vi "HEWH Extract DBL Data.vi"(7 "Full Data (String)":string[][](array[string]), 8 "error in (no error)":errorcluster, 10 "Full Data DBL In":dbl[][](array[numeric]), 11 "UEF Calculated Values Input in":T1 {"Data Indexes"."15 sec after Draw Index" format="%#.2f"; "Data Indexes"."15 sec after Draw Timestamp" format="%#.2f"; "Data Indexes"."Test Start Timestamp" format="%.2f"; "Data Indexes"."Test End Timestamp" format="%.2f"; "Data Indexes"."T0 Timestamp" format="%.2f"; "Data Indexes"."Tsf Timestamp" format="%.2f"; "Data Indexes"."Tsu0 Timestamp" format="%.2f"; "Data Indexes"."Tmax1 Timestamp" format="%.2f"; "Data Indexes"."Draw Index Timestamp" format="%#.2f"; "Data Indexes"."Non-Draw Timestamp" format="%#.2f"; "Data Indexes"."Heating Timestamp" format="%#.2f"; "Data Indexes"."Start Energy (BTU-Gas)" format="%.6f"; "Data Indexes"."Start Watt Hours" format="%.6f"; "Static Data"."V - Volume of Wh (True)" format="%.5f"; "Static Data"."T-Ambinet Nominal (°F)" format="%.5f"; "Static Data"."T-Inlet Setpoint (°F)" format="%.5f"; "Static Data"."T-Wh Setpoint (°F)" format="%.5f"; "Sampled Data"."Qe (Wh)" format="%.5f"; "Sampled Data"."Tau stby2 (hr)" format="%.5f"; "Sampled Data"."Tastby2 (°F)" format="%.5f"; "Sampled Data"."Qf (BTU)" format="%.5f"; "Sampled Data"."Qe (BTU)" format="%.5f"; "Sampled Data"."Tmax1 (°F)" format="%.5f"; "Sampled Data"."T0 (°F)" format="%.5f"; "Sampled Data"."Qr (BTU)" format="%.5f"; "Sampled Data"."T 24(°F)" format="%.5f"; "Sampled Data"."T astby(°F)" format="%.5f"; "Sampled Data"."T tstby(°F)" format="%.5f"; "Sampled Data"."T su0(°F)" format="%.5f"; "Sampled Data"."T suf(°F)" format="%.5f"; "Sampled Data"."Tau stby_1 (hr)" format="%.5f"; "Sampled Data"."Qsuf (BTU)" format="%.5f"; "Sampled Data"."Qsu0 (BTU)" format="%.5f"; "Calculated Values"."Draw Bonus Volume (gal)" format="%.6f"; "Calculated Values"."Adjustment Factor" format="%.6f"; "Calculated Values"."T*avg_del(n-1)" format="%.6f"; "Calculated Values"."T*min(n-1)" format="%.6f"; "Calculated Values"."T*avg_del(n)" format="%.6f"; "Calculated Values"."Vn" format="%.6f"; "Calculated Values"."Qdm (BTU)" format="%.6f"; "Calculated Values"."QHWD (BTU)" format="%.6f"; "Calculated Values"."QHW (BTU)" format="%.6f"; "Calculated Values"."UEF" format="%.6f"; "Calculated Values"."QHW67 (BTU)" format="%.6f"; "Calculated Values"."Qda (BTU)" format="%.6f"; "Calculated Values"."Qd (BTU)" format="%.6f"; "Calculated Values"."Q (BTU)" format="%.6f"; "Calculated Values"."UA (BTU/(hr*F))" format="%.6f"; "Calculated Values"."Qhr (BTU/hr)" format="%.6f"; "Calculated Values"."Qstby (BTU)" format="%.6f"; "Calculated Values"."nu_r" format="%.6f"; "Calculated Values"."CpUEF (BTU/(lb*F))" format="%.6f"; "Calculated Values"."rho_nu (lb/gal)" format="%.6f"; "Calculated Values"."V1- Vol (Gal)" format="%.6f"; "Calculated Values"."M cluster mass removed (lb)" format="%.6f"; "Calculated Values"."Cp theoretical (BTU/(lbm °F))" format="%.6f"; "Calculated Values"."Tin1 - Mean Inlet 1st Cluster (°F)" format="%.6f"; "Calculated Values"."Tdel1-Mean Outlet 1st Cluster(°F)" format="%.6f"; "Calculated Values"."Cp 24 (BTU/(lb*F))" format="%.6f"; "Calculated Values"."Cp standby (BTU/(lb*F))" format="%.6f"; "Calculated Values"."Cp2 (BTU/(lb*F))" format="%.6f"; "Calculated Values"."Cp1 (BTU/(lb*F))" format="%.6f"; "Calculated Values"."rho 24 (lb/gal)" format="%.6f"; "Calculated Values"."rho standby (lb/gal)" format="%.6f"; "Calculated Values"."rho 2 (lb/gal)" format="%.6f"; "Calculated Values"."Density of cold water All (lbm/gal)" format="%#.3g"; "Calculated Values"."CpHW (BTU/(lbm °F))" format="%#.3g"; "Calculated Values"."Density of hot water All (lbm/gal)" format="%#.3g"; "Calculated Values"."Mass of water All (lbm)" format="%#.3f"}) -> (0 "error out":errorcluster, 2 "Full Data DBL Out":dbl[][](array[numeric]), 3 "UEF Calculated Values Input out":T1 {"Data Indexes"."15 sec after Draw Index" format="%#.2f"; "Data Indexes"."15 sec after Draw Timestamp" format="%#.2f"; "Data Indexes"."Test Start Timestamp" format="%.2f"; "Data Indexes"."Test End Timestamp" format="%.2f"; "Data Indexes"."T0 Timestamp" format="%.2f"; "Data Indexes"."Tsf Timestamp" format="%.2f"; "Data Indexes"."Tsu0 Timestamp" format="%.2f"; "Data Indexes"."Tmax1 Timestamp" format="%.2f"; "Data Indexes"."Draw Index Timestamp" format="%#.2f"; "Data Indexes"."Non-Draw Timestamp" format="%#.2f"; "Data Indexes"."Heating Timestamp" format="%#.2f"; "Data Indexes"."Start Energy (BTU-Gas)" format="%.6f"; "Data Indexes"."Start Watt Hours" format="%.6f"; "Static Data"."V - Volume of Wh (True)" format="%.5f"; "Static Data"."T-Ambinet Nominal (°F)" format="%.5f"; "Static Data"."T-Inlet Setpoint (°F)" format="%.5f"; "Static Data"."T-Wh Setpoint (°F)" format="%.5f"; "Sampled Data"."Qe (Wh)" format="%.5f"; "Sampled Data"."Tau stby2 (hr)" format="%.5f"; "Sampled Data"."Tastby2 (°F)" format="%.5f"; "Sampled Data"."Qf (BTU)" format="%.5f"; "Sampled Data"."Qe (BTU)" format="%.5f"; "Sampled Data"."Tmax1 (°F)" format="%.5f"; "Sampled Data"."T0 (°F)" format="%.5f"; "Sampled Data"."Qr (BTU)" format="%.5f"; "Sampled Data"."T 24(°F)" format="%.5f"; "Sampled Data"."T astby(°F)" format="%.5f"; "Sampled Data"."T tstby(°F)" format="%.5f"; "Sampled Data"."T su0(°F)" format="%.5f"; "Sampled Data"."T suf(°F)" format="%.5f"; "Sampled Data"."Tau stby_1 (hr)" format="%.5f"; "Sampled Data"."Qsuf (BTU)" format="%.5f"; "Sampled Data"."Qsu0 (BTU)" format="%.5f"; "Calculated Values"."Draw Bonus Volume (gal)" format="%.6f"; "Calculated Values"."Adjustment Factor" format="%.6f"; "Calculated Values"."T*avg_del(n-1)" format="%.6f"; "Calculated Values"."T*min(n-1)" format="%.6f"; "Calculated Values"."T*avg_del(n)" format="%.6f"; "Calculated Values"."Vn" format="%.6f"; "Calculated Values"."Qdm (BTU)" format="%.6f"; "Calculated Values"."QHWD (BTU)" format="%.6f"; "Calculated Values"."QHW (BTU)" format="%.6f"; "Calculated Values"."UEF" format="%.6f"; "Calculated Values"."QHW67 (BTU)" format="%.6f"; "Calculated Values"."Qda (BTU)" format="%.6f"; "Calculated Values"."Qd (BTU)" format="%.6f"; "Calculated Values"."Q (BTU)" format="%.6f"; "Calculated Values"."UA (BTU/(hr*F))" format="%.6f"; "Calculated Values"."Qhr (BTU/hr)" format="%.6f"; "Calculated Values"."Qstby (BTU)" format="%.6f"; "Calculated Values"."nu_r" format="%.6f"; "Calculated Values"."CpUEF (BTU/(lb*F))" format="%.6f"; "Calculated Values"."rho_nu (lb/gal)" format="%.6f"; "Calculated Values"."V1- Vol (Gal)" format="%.6f"; "Calculated Values"."M cluster mass removed (lb)" format="%.6f"; "Calculated Values"."Cp theoretical (BTU/(lbm °F))" format="%.6f"; "Calculated Values"."Tin1 - Mean Inlet 1st Cluster (°F)" format="%.6f"; "Calculated Values"."Tdel1-Mean Outlet 1st Cluster(°F)" format="%.6f"; "Calculated Values"."Cp 24 (BTU/(lb*F))" format="%.6f"; "Calculated Values"."Cp standby (BTU/(lb*F))" format="%.6f"; "Calculated Values"."Cp2 (BTU/(lb*F))" format="%.6f"; "Calculated Values"."Cp1 (BTU/(lb*F))" format="%.6f"; "Calculated Values"."rho 24 (lb/gal)" format="%.6f"; "Calculated Values"."rho standby (lb/gal)" format="%.6f"; "Calculated Values"."rho 2 (lb/gal)" format="%.6f"; "Calculated Values"."Density of cold water All (lbm/gal)" format="%#.3g"; "Calculated Values"."CpHW (BTU/(lbm °F))" format="%#.3g"; "Calculated Values"."Density of hot water All (lbm/gal)" format="%#.3g"; "Calculated Values"."Mass of water All (lbm)" format="%#.3f"})   [LabVIEW 2023]
uses:
  Type Definitions/UEF Constants.ctl
  Type Definitions/HEWH Draw Stats.ctl
  Type Definitions/HEWH FHR Draw Type.ctl
  Type Definitions/FHR Bins.ctl
  Type Definitions/HEWH Meter Type.ctl
panel:
  # "FHR"
  # "FHR"
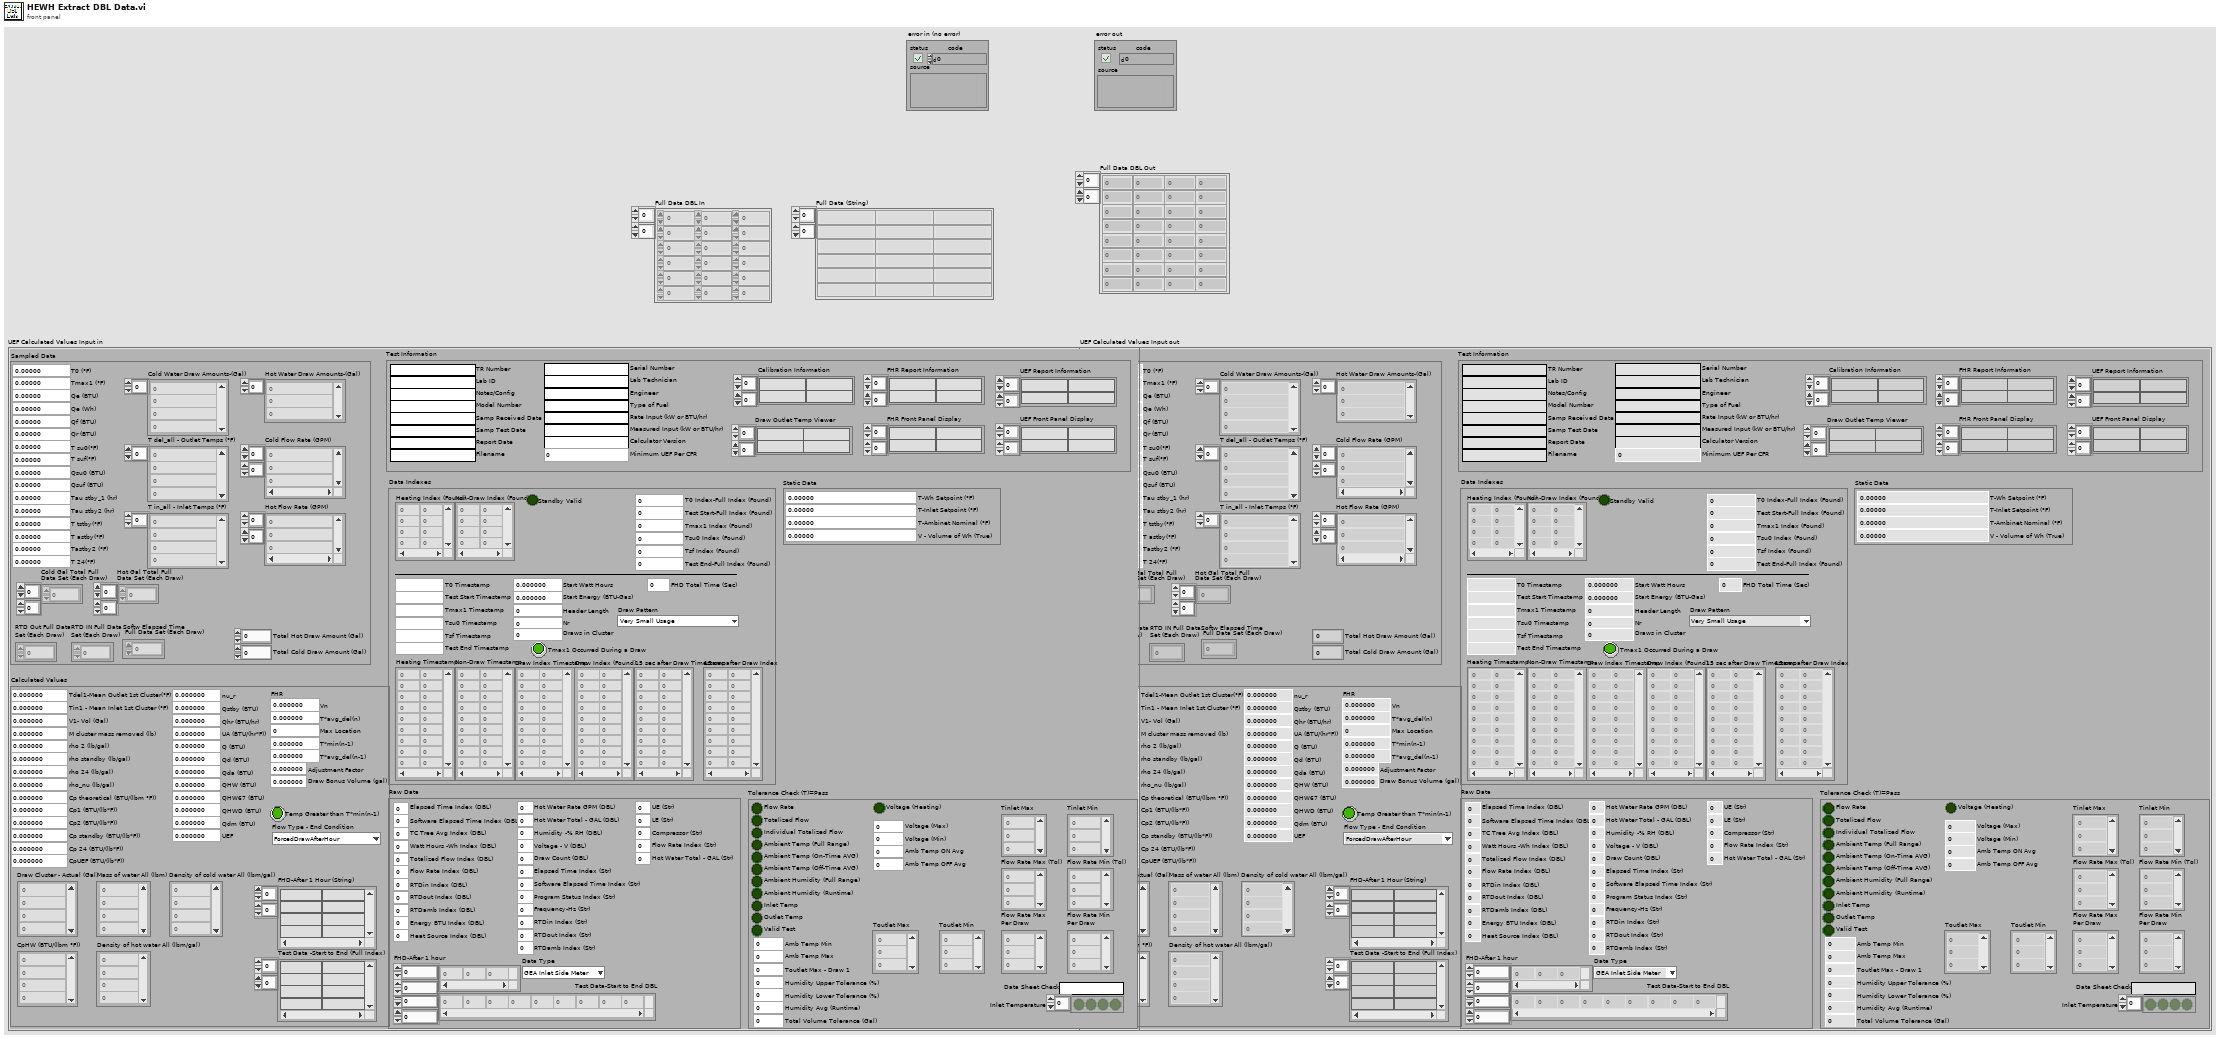
[diagram p1: front panel]
types:
  T1 = typedef "UEF Constants.ctl" = cluster{"Calculated Values":T2, "Sampled Data":cluster{"Cold Water Draw Amounts-(Gal)":dbl[], "T del_all - Outlet Temps (°F)":dbl[], "T in_all - Inlet Temps (°F)":dbl[], "Qsu0 (BTU)":dbl, "Qsuf (BTU)":dbl, "Tau stby_1 (hr)":dbl, "T suf(°F)":dbl, "T su0(°F)":dbl, "T tstby(°F)":dbl, "T astby(°F)":dbl, "T 24(°F)":dbl, "Qr (BTU)":dbl, "T0 (°F)":dbl, "Tmax1 (°F)":dbl, "Qe (BTU)":dbl, "Qf (BTU)":dbl, "Tastby2 (°F)":dbl, "RTD Out Full Data\nSet (Each Draw)":dbl[][], "RTD IN Full Data\nSet (Each Draw)":dbl[][], "Tau stby2 (hr)":dbl, "Hot Water Draw Amounts-(Gal)":dbl[], "Cold Flow Rate (GPM)":dbl[][], "Hot Flow Rate (GPM)":dbl[][], "Softw Elapsed Time\n Full Data Set (Each Draw)":dbl[][], "Cold Gal Total Full\nData Set (Each Draw)":dbl[][], "Total Hot Draw Amount (Gal) ":dbl, "Total Cold Draw Amount (Gal)":dbl, "Qe (Wh)":dbl, "Hot Gal Total Full\nData Set (Each Draw)":dbl[][]}, "Static Data":cluster{"T-Wh Setpoint (°F)":dbl, "T-Inlet Setpoint (°F)":dbl, "T-Ambinet Nominal (°F)":dbl, "V - Volume of Wh (True)":dbl}, "Data Indexes":cluster{"Test Start-Full Index (Found)":i32, "Header Length":i32, "Draw Index (Found)":i32[][], "Nr":i32, "Start Watt Hours":dbl, "Tsu0 Index (Found)":i32, "Tsf Index (Found)":i32, "Start Energy (BTU-Gas)":dbl, "Draws in Cluster":i32, "T0 Index-Full Index (Found)":i32, "Non-Draw Index (Found)":i32[][], "Tmax1 Index (Found)":i32, "Test End-Full Index (Found)":i32, "Heating Index (Found)":i32[][], "Heating Timestamp":dbl[][], "Non-Draw Timestamp":dbl[][], "Draw Index Timestamp":dbl[][], "Tmax1 Timestamp":dbl, "Tsu0 Timestamp":dbl, "Tsf Timestamp":dbl, "T0 Timestamp":dbl, "Test End Timestamp":dbl, "Test Start Timestamp":dbl, "15 sec after Draw Timestamp":dbl[][], "15 sec after Draw Index":dbl[][], "Tmax1 Occurred During a Draw":bool, "FHD Total Time (Sec)":dbl, "Draw Pattern":T4, "Standby Valid":bool}, "Raw Data":cluster{"Elapsed Time Index (DBL)":i32, "Software Elapsed Time Index (DBL)":i32, "TC Tree Avg Index (DBL)":i32, "Watt Hours -Wh Index (DBL)":i32, "Energy BTU Index (DBL)":i32, "Totalized Flow Index (DBL)":i32, "Flow Rate Index (DBL)":i32, "Program Status Index (Str)":i32, "RTDin Index (DBL)":i32, "RTDout Index (DBL)":i32, "RTDamb Index (DBL)":i32, "Test Data-Start to End DBL":dbl[][], "Data Type":T5, "Heat Source Index (DBL)":i32, "Hot Water Rate GPM (DBL)":i32, "Hot Water Total - GAL (DBL)":i32, "FHD-After 1 hour":dbl[][], "Humidity -% RH (DBL)":i32, "Voltage - V (DBL)":i32, "Draw Count (DBL)":i32, "Elapsed Time Index (Str)":i32, "Software Elapsed Time Index (Str)":i32, "Frequency-Hz (Str)":i32, "RTDin Index (Str)":i32, "RTDout Index (Str)":i32, "RTDamb Index (Str)":i32, "UE (Str)":i32, "LE (Str)":i32, "Compressor (Str)":i32, "Flow Rate Index (Str)":i32, "Hot Water Total - GAL (Str)":i32}, "Tolerance Check (T)=Pass":cluster{"Flow Rate":bool, "Totalized Flow":bool, "Ambient Temp (Full Range)":bool, "Ambient Humidity (Full Range)":bool, "Inlet Temp":bool, "Outlet Temp":bool, "Valid Test":bool, "Individual Totalized Flow":bool, "Data Sheet Check":string, "Inlet Temperature":bool[], "Tinlet Max":dbl[], "Tinlet Min":dbl[], "Flow Rate Max (Tol)":dbl[], "Flow Rate Min (Tol)":dbl[], "Amb Temp Max":dbl, "Amb Temp Min":dbl, "Toutlet Max - Draw 1":dbl, "Humidity Upper Tolerance (%)":dbl, "Total Volume Tolerance (Gal)":dbl, "Humidity Lower Tolerance (%)":dbl, "Flow Rate Max\nPer Draw":dbl[], "Flow Rate Min\nPer Draw":dbl[], "Ambient Humidity (Runtime)":bool, "Humidity Avg (Runtime)":dbl, "Ambient Temp (On-Time AVG)":bool, "Ambient Temp (Off-Time AVG)":bool, "Amb Temp OFF Avg":dbl, "Amb Temp ON Avg":dbl, "Voltage (Heating)":bool, "Voltage (Min)":dbl, "Voltage (Max)":dbl, "Toutlet Max":dbl[], "Toutlet Min":dbl[]}, "Test Information":cluster{"TR Number":string, "Lab ID":string, "Notes/Config":string, "Model Number":string, "Serial Number":string, "Lab Technician":string, "Engineer":string, "Type of Fuel":string, "Samp Received Date":string, "Samp Test Date":string, "Report Date":string, "Rate Input (kW or BTU/hr)":string, "Measured Input (kW or BTU/hr)":string, "Filename":string, "Calibration Information":string[][], "Calculator Version":string, "Minimum UEF Per CFR":dbl, "UEF Report Information":string[][], "FHR Report Information":string[][], "FHR Front Panel Display":string[][], "UEF Front Panel Display":string[][], "Draw Outlet Temp Viewer":string[][]}}
  T2 = typedef "HEWH Draw Stats.ctl" = cluster{"Draw Cluster - Actual (Gal)":dbl[], "Mass of water All (lbm)":dbl[], "Density of hot water All (lbm/gal)":dbl[], "CpHW (BTU/(lbm °F))":dbl[], "rho 2 (lb/gal)":dbl, "rho standby (lb/gal)":dbl, "rho 24 (lb/gal)":dbl, "Cp1 (BTU/(lb*F))":dbl, "Cp2 (BTU/(lb*F))":dbl, "Cp standby (BTU/(lb*F))":dbl, "Cp 24 (BTU/(lb*F))":dbl, "nu_r":dbl, "Qstby (BTU)":dbl, "Qhr (BTU/hr)":dbl, "UA (BTU/(hr*F))":dbl, "Q (BTU)":dbl, "Qd (BTU)":dbl, "Qda (BTU)":dbl, "QHW67 (BTU)":dbl, "UEF":dbl, "Tdel1-Mean Outlet 1st Cluster(°F)":dbl, "Tin1 - Mean Inlet 1st Cluster (°F)":dbl, "Cp theoretical (BTU/(lbm °F))":dbl, "M cluster mass removed (lb)":dbl, "V1- Vol (Gal)":dbl, "Test Data -Start to End (Full Index)":string[][], "rho_nu (lb/gal)":dbl, "Density of cold water All (lbm/gal)":dbl[], "CpUEF (BTU/(lb*F))":dbl, "QHW (BTU)":dbl, "QHWD (BTU)":dbl, "Qdm (BTU)":dbl, "FHD-After 1 Hour (String)":string[][], "Vn":dbl, "T*avg_del(n)":dbl, "Max Location":i32, "T*min(n-1)":dbl, "T*avg_del(n-1)":dbl, "Temp Greater than T*min(n-1)":bool, "Adjustment Factor":dbl, "Draw Bonus Volume (gal)":dbl, "Flow Type - End Condition":T3}
  T3 = typedef "HEWH FHR Draw Type.ctl" = enum16{"ForcedDrawAfterHour", "HeatingCutoffBeforeHour"}
  T4 = typedef "FHR Bins.ctl" = enum16{"Very Small Usage", "Low Usage", "Medium Usage", "High Usage", "Undefined"}
  T5 = typedef "HEWH Meter Type.ctl" = enum16{"GEA Inlet Side Meter", "GEA Outlet Side Meter", "CSA Inlet Side Meter"}
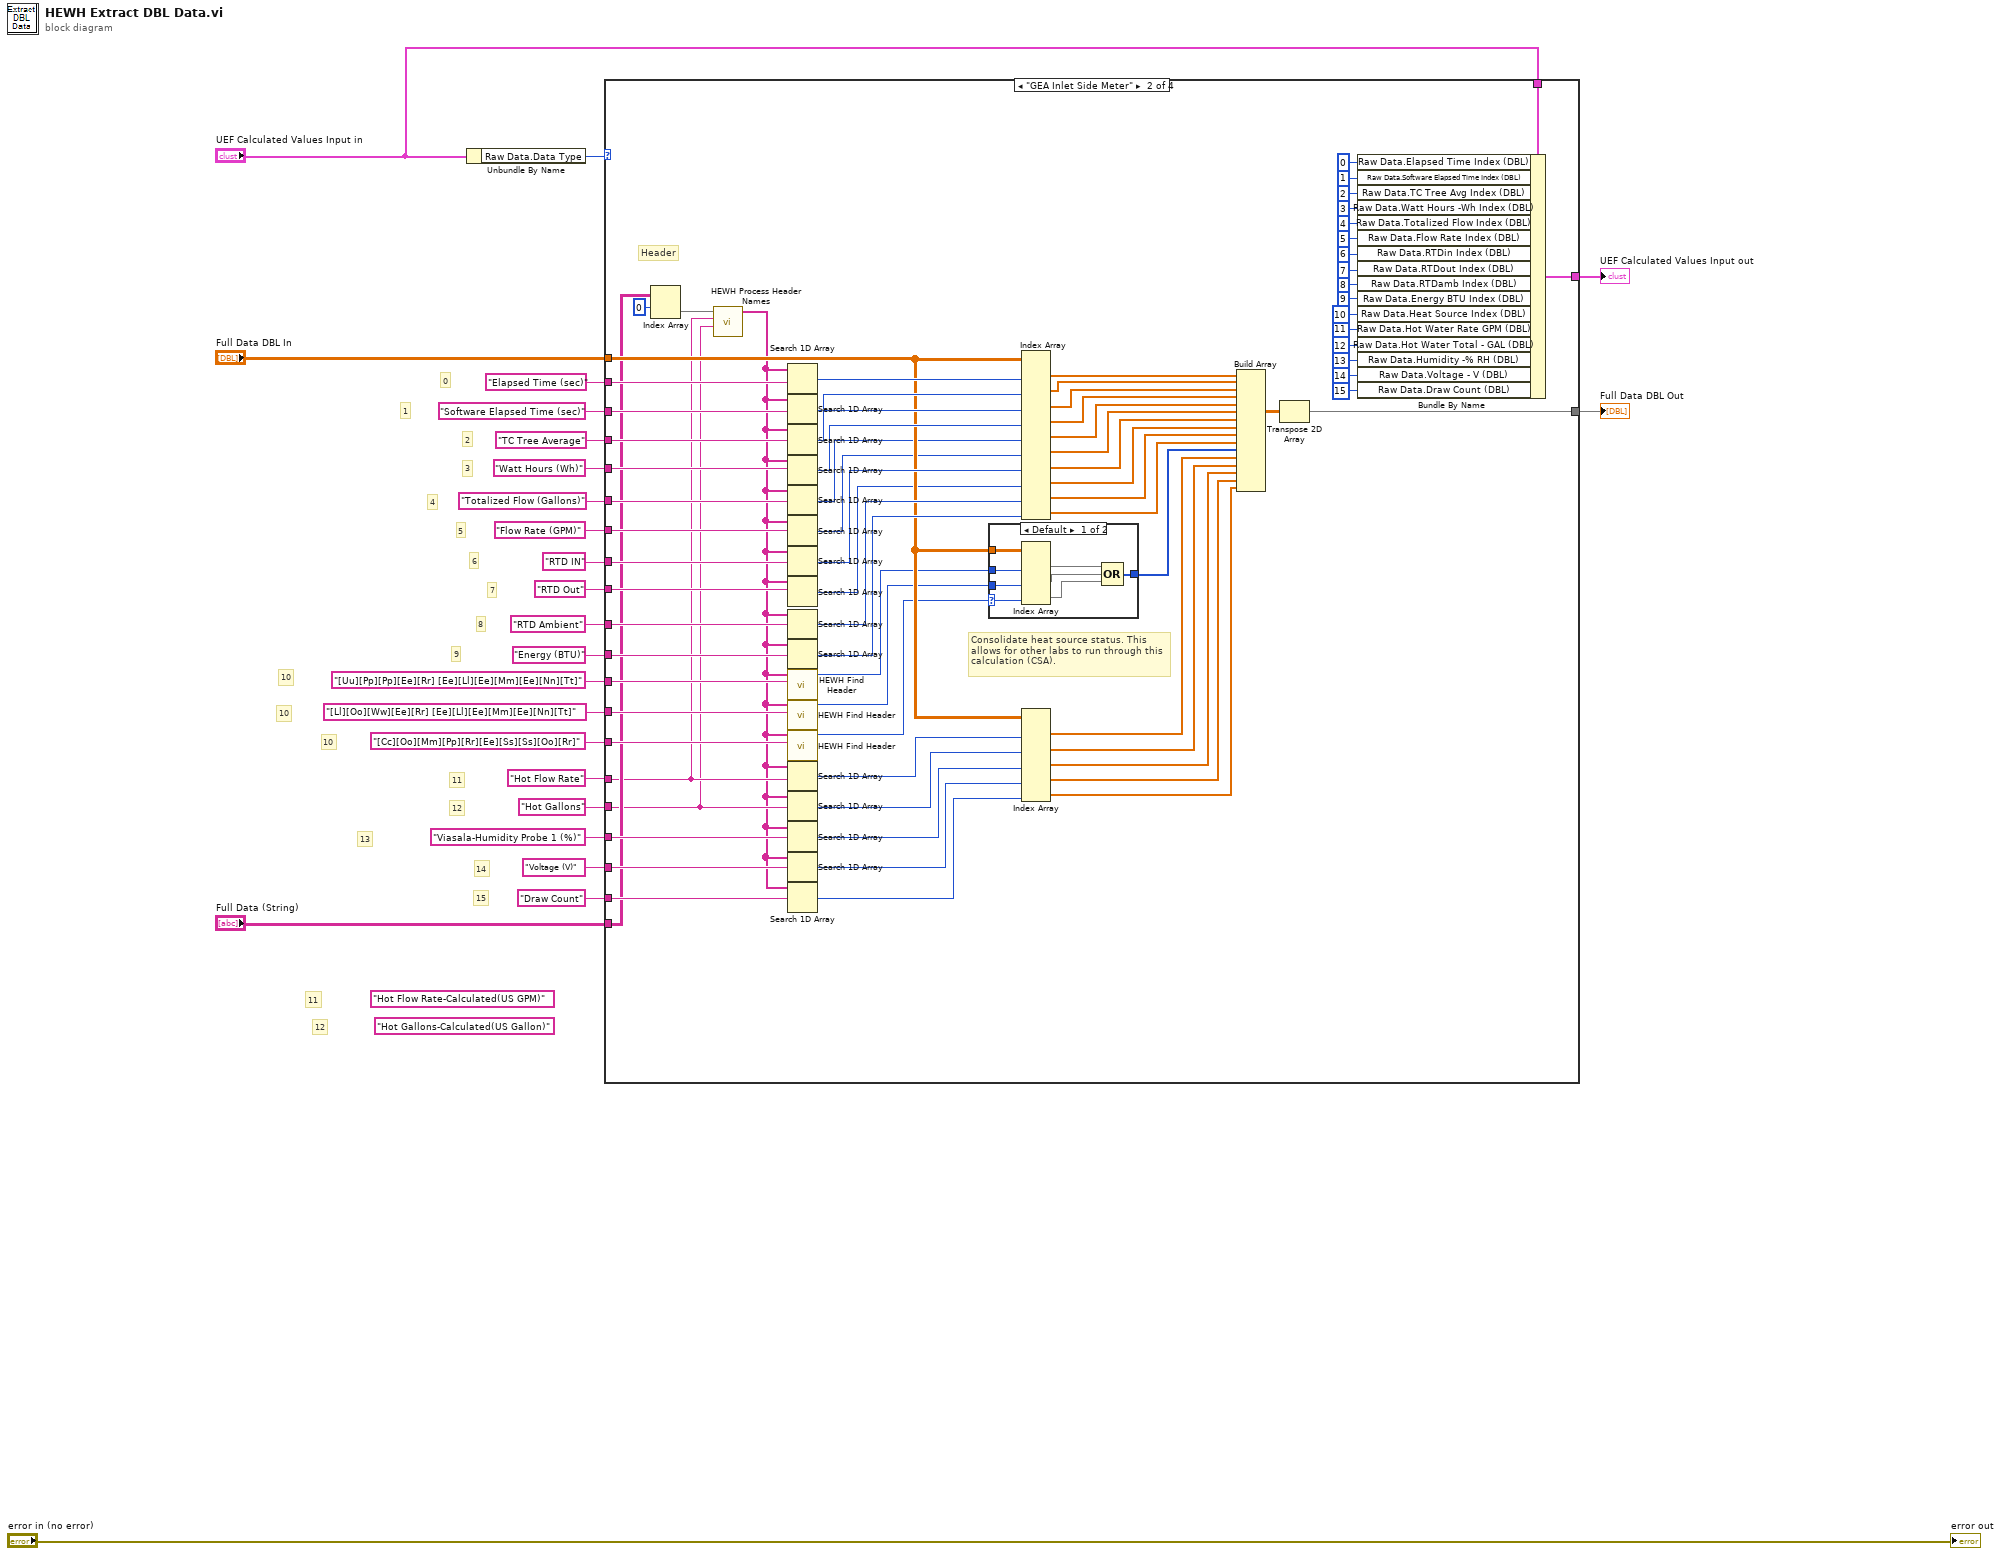
[diagram p0: block diagram]
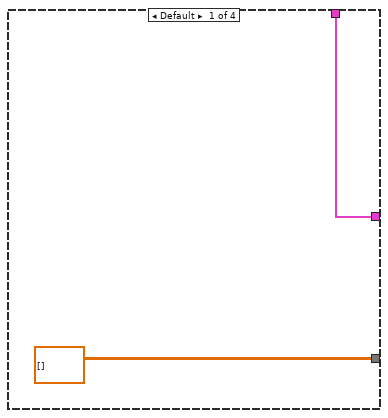
[diagram p2: hidden frame]
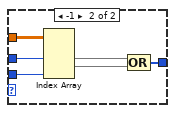
[diagram p3: hidden frame]
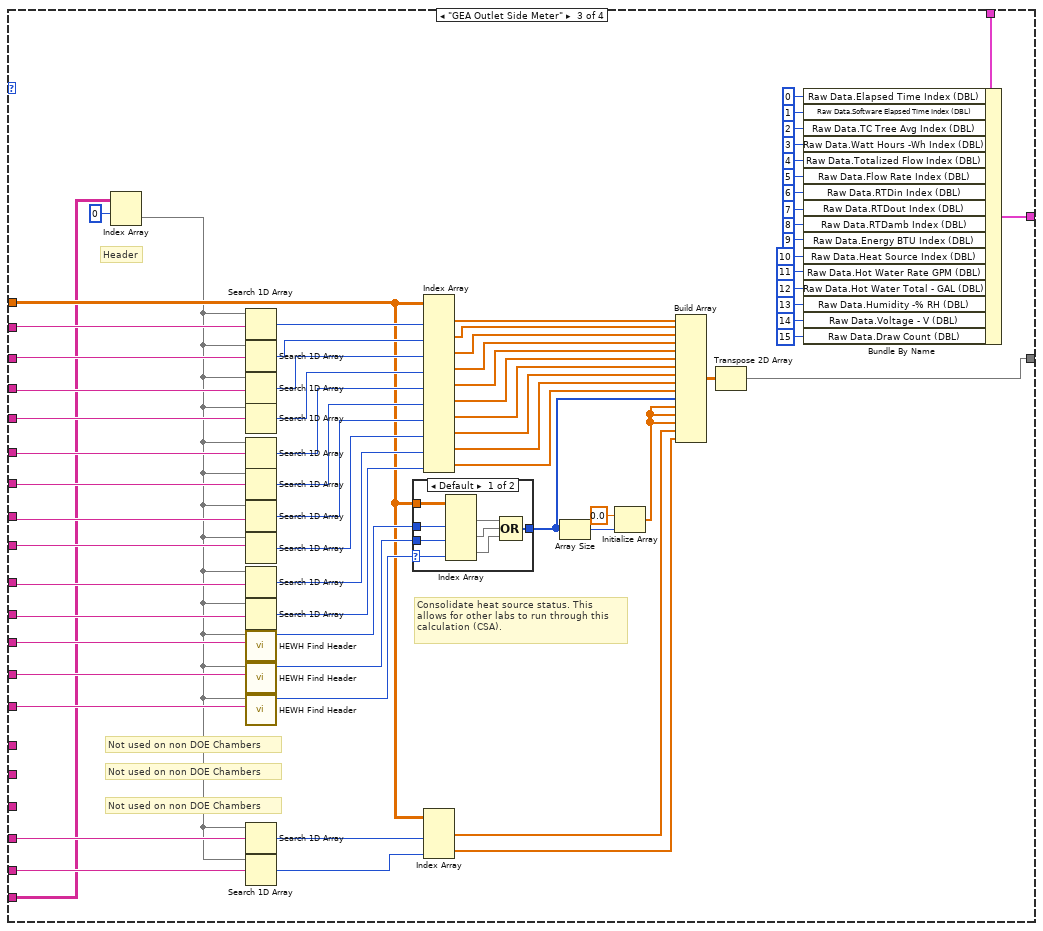
[diagram p4: hidden frame]
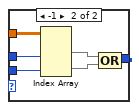
[diagram p5: hidden frame]
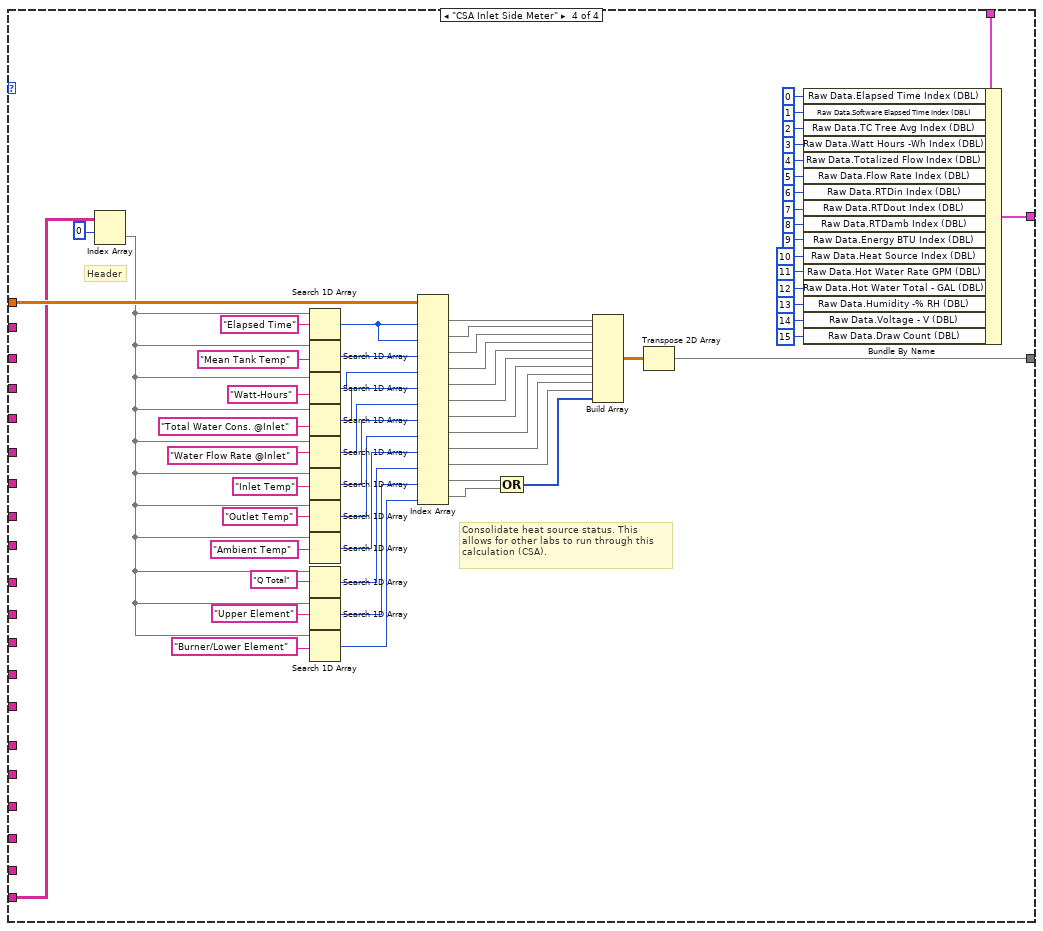
[diagram p6: hidden frame]
diagram:
  (unwired) "Hot Gallons-Calculated(US Gallon)" ("regular expression")
  (unwired) "Hot Flow Rate-Calculated(US GPM)" ("regular expression")
  # "12"
  # "11"
  # "15"
  # "14"
  # "13"
  # "12"
  # "11"
  # "10"
  # "10"
  # "10"
  # "9"
  # "8"
  # "7"
  # "6"
  # "5"
  # "4"
  # "3"
  # "2"
  # "1"
  # "0"
  n1 = Unbundle By Name("UEF Calculated Values Input in") -> ("Raw Data.Data Type"=w3:T5)
  n2 = case shown="\"GEA Inlet Side Meter\"" w3 {
    tunnel: [dbl[][] [] w104 w167 w260] -> w24
    tunnel: "Full Data DBL In" -> [_ w81 w144 w261]
    tunnel: "Full Data (String)" -> [_ w32 w119 w204]
    tunnel: "Elapsed Time (sec)" ("regular expression") -> [_ w67 w163 _]
    tunnel: "Software Elapsed Time (sec)" ("regular expression") -> [_ w66 w162 _]
    tunnel: "TC Tree Average" ("regular expression") -> [_ w65 w161 _]
    tunnel: "Watt Hours (Wh)" ("regular expression") -> [_ w64 w160 _]
    tunnel: "Totalized Flow (Gallons)" ("regular expression") -> [_ w63 w159 _]
    tunnel: "Flow Rate (GPM)" ("regular expression") -> [_ w62 w158 _]
    tunnel: "RTD IN" ("regular expression") -> [_ w61 w157 _]
    tunnel: "RTD Out" ("regular expression") -> [_ w60 w156 _]
    tunnel: "RTD Ambient" ("regular expression") -> [_ w59 w155 _]
    tunnel: "Energy (BTU)" ("regular expression") -> [_ w58 w154 _]
    tunnel: "[Uu][Pp][Pp][Ee][Rr] [Ee][Ll][Ee][Mm][Ee][Nn][Tt]" ("Expression") -> [_ w57 w153 _]
    tunnel: "[Ll][Oo][Ww][Ee][Rr] [Ee][Ll][Ee][Mm][Ee][Nn][Tt]" ("regular expression") -> [_ w56 w152 _]
    tunnel: "[Cc][Oo][Mm][Pp][Rr][Ee][Ss][Ss][Oo][Rr]" ("regular expression") -> [_ w55 w151 _]
    tunnel: "Hot Flow Rate" ("regular expression") -> [_ w31 _ _]
    tunnel: "Hot Gallons" ("regular expression") -> [_ w30 _ _]
    tunnel: "Viasala-Humidity Probe 1 (%)" ("regular expression") -> [_ w54 _ _]
    tunnel: "Voltage (V)" ("regular expression") -> [_ w53 w146 _]
    tunnel: "Draw Count" ("regular expression") -> [_ w52 w145 _]
    tunnel: "UEF Calculated Values Input in" -> [w26 w35 w123 w207]
    tunnel: [w26 w34 w122 w206] -> w25
    frame Default {
    }
    frame "GEA Inlet Side Meter" {
      # "Header"
      # "Consolidate heat source status. This \nallows for other labs to run through this\ncalculation (CSA)."
      n3 = Index Array(array=w32, index (row)=0) -> (element=w29:string[])  [unwired: 1 in]
      n4 = call "HEWH Process Header Names.vi"("Search Expression 2"=w30, "Search Expression 1"=w31, "Header"=w29) -> ("Output Header"=w28:string[])  [unwired: 8 in]
      n5 = Search 1D Array(1D array=w28, element=w67) -> (index of element=w94:i32)  [unwired: 1 in]
      n6 = Search 1D Array(1D array=w28, element=w66) -> (index of element=w95:i32)  [unwired: 1 in]
      n7 = Search 1D Array(1D array=w28, element=w65) -> (index of element=w96:i32)  [unwired: 1 in]
      n8 = Search 1D Array(1D array=w28, element=w64) -> (index of element=w84:i32)  [unwired: 1 in]
      n9 = Search 1D Array(1D array=w28, element=w63) -> (index of element=w76:i32)  [unwired: 1 in]
      n10 = Search 1D Array(1D array=w28, element=w62) -> (index of element=w77:i32)  [unwired: 1 in]
      n11 = Search 1D Array(1D array=w28, element=w61) -> (index of element=w83:i32)  [unwired: 1 in]
      n12 = Search 1D Array(1D array=w28, element=w60) -> (index of element=w74:i32)  [unwired: 1 in]
      n13 = Search 1D Array(1D array=w28, element=w59) -> (index of element=w82:i32)  [unwired: 1 in]
      n14 = Search 1D Array(1D array=w28, element=w58) -> (index of element=w89:i32)  [unwired: 1 in]
      n15 = call "HEWH Find Header.vi"("Expression"=w57, "Header"=w28) -> ("Index"=w80:i32)  [unwired: 9 in]
      n16 = call "HEWH Find Header.vi"("Expression"=w56, "Header"=w28) -> ("Index"=w79:i32)  [unwired: 9 in]
      n17 = call "HEWH Find Header.vi"("Expression"=w55, "Header"=w28) -> ("Index"=w78:i32)  [unwired: 9 in]
      n18 = Search 1D Array(1D array=w28, element=w31) -> (index of element=w87:i32)  [unwired: 1 in]
      n19 = Search 1D Array(1D array=w28, element=w30) -> (index of element=w75:i32)  [unwired: 1 in]
      n20 = Search 1D Array(1D array=w28, element=w54) -> (index of element=w73:i32)  [unwired: 1 in]
      n21 = Search 1D Array(1D array=w28, element=w53) -> (index of element=w71:i32)  [unwired: 1 in]
      n22 = Search 1D Array(1D array=w28, element=w52) -> (index of element=w69:i32)  [unwired: 1 in]
      n23 = case shown="Default" w78 {
        selector: w78 -> [w108 _]
        tunnel: [w112 w115] -> w88
        tunnel: w81 -> [w111 w116]
        tunnel: w80 -> [w110 w114]
        tunnel: w79 -> [w109 w113]
        frame Default {
          n24 = Index Array(array=w111, index (col) #1=w110, index (col) #2=w109, index (col) #3=w108) -> (element #1=w107:dbl[], element #2=w106:dbl[], element #3=w105:dbl[])  [unwired: 3 in]
          n25 = Compound Arithmetic op=OR(w107, w106, w105) -> (w112:i32[])
        }
        frame -1 {
          n26 = Index Array(array=w116, index (col) #1=w114, index (col) #2=w113) -> (element #1=w118:dbl[], element #2=w117:dbl[])  [unwired: 2 in]
          n27 = Compound Arithmetic op=OR(w118, w117) -> (w115:i32[])
        }
      }
      n28 = Index Array(array=w81, index (col) #1=w94, index (col) #2=w95, index (col) #3=w96, index (col) #4=w84, index (col) #5=w76, index (col) #6=w77, index (col) #7=w83, index (col) #8=w74, index (col) #9=w82, index (col) #10=w89) -> (element #1=w102:dbl[], element #2=w97:dbl[], element #3=w98:dbl[], element #4=w99:dbl[], element #5=w100:dbl[], element #6=w101:dbl[], element #7=w93:dbl[], element #8=w92:dbl[], element #9=w91:dbl[], element #10=w90:dbl[])  [unwired: 10 in]
      n29 = Index Array(array=w81, index (col) #1=w87, index (col) #2=w75, index (col) #3=w73, index (col) #4=w71, index (col) #5=w69) -> (element #1=w86:dbl[], element #2=w85:dbl[], element #3=w72:dbl[], element #4=w70:dbl[], element #5=w68:dbl[])  [unwired: 5 in]
      n30 = Build Array(w102, w97, w98, w99, w100, w101, w93, w92, w91, w90, w88, w86, w85, w72, w70, w68) -> (w103:dbl[][])
      n31 = Transpose 2D Array(2D array=w103) -> (transposed array=w104:dbl[][])
      n32 = Bundle By Name(cluster=w35, "Raw Data.Elapsed Time Index (DBL)"=0 ("Raw Data.Elapsed Time Index"), "Raw Data.Software Elapsed Time Index (DBL)"=1 ("Raw Data.Elapsed Time Index"), "Raw Data.TC Tree Avg Index (DBL)"=2 ("Raw Data.Elapsed Time Index"), "Raw Data.Watt Hours -Wh Index (DBL)"=3 ("Raw Data.Elapsed Time Index"), "Raw Data.Totalized Flow Index (DBL)"=4 ("Raw Data.Elapsed Time Index"), "Raw Data.Flow Rate Index (DBL)"=5 ("Raw Data.Elapsed Time Index"), "Raw Data.RTDin Index (DBL)"=6 ("Raw Data.Elapsed Time Index"), "Raw Data.RTDout Index (DBL)"=7 ("Raw Data.Elapsed Time Index"), "Raw Data.RTDamb Index (DBL)"=8 ("Raw Data.Elapsed Time Index"), "Raw Data.Energy BTU Index (DBL)"=9 ("Raw Data.Elapsed Time Index"), "Raw Data.Heat Source Index (DBL)"=10 ("Raw Data.Elapsed Time Index"), "Raw Data.Hot Water Rate GPM (DBL)"=11 ("Raw Data.Elapsed Time Index"), "Raw Data.Hot Water Total - GAL (DBL)"=12 ("Raw Data.Elapsed Time Index"), "Raw Data.Humidity -% RH (DBL)"=13 ("Raw Data.Elapsed Time Index"), "Raw Data.Voltage - V (DBL)"=14 ("Raw Data.Elapsed Time Index"), "Raw Data.Draw Count (DBL)"=15 ("Raw Data.Elapsed Time Index")) -> (w34:T1)
    }
    frame "GEA Outlet Side Meter" {
      # "Header"
      # "Not used on non DOE Chambers"
      # "Not used on non DOE Chambers"
      # "Not used on non DOE Chambers"
      # "Consolidate heat source status. This \nallows for other labs to run through this\ncalculation (CSA)."
      n33 = Index Array(array=w119, index (row)=0) -> (element=w120:string[])  [unwired: 1 in]
      n34 = Search 1D Array(1D array=w120, element=w163) -> (index of element=w176:i32)  [unwired: 1 in]
      n35 = Search 1D Array(1D array=w120, element=w162) -> (index of element=w177:i32)  [unwired: 1 in]
      n36 = Search 1D Array(1D array=w120, element=w161) -> (index of element=w178:i32)  [unwired: 1 in]
      n37 = Search 1D Array(1D array=w120, element=w160) -> (index of element=w179:i32)  [unwired: 1 in]
      n38 = Search 1D Array(1D array=w120, element=w159) -> (index of element=w180:i32)  [unwired: 1 in]
      n39 = Search 1D Array(1D array=w120, element=w158) -> (index of element=w181:i32)  [unwired: 1 in]
      n40 = Search 1D Array(1D array=w120, element=w157) -> (index of element=w166:i32)  [unwired: 1 in]
      n41 = Search 1D Array(1D array=w120, element=w156) -> (index of element=w165:i32)  [unwired: 1 in]
      n42 = Search 1D Array(1D array=w120, element=w155) -> (index of element=w164:i32)  [unwired: 1 in]
      n43 = Search 1D Array(1D array=w120, element=w154) -> (index of element=w171:i32)  [unwired: 1 in]
      n44 = call "HEWH Find Header.vi"("Expression"=w153, "Header"=w120) -> ("Index"=w169:i32)  [unwired: 9 in]
      n45 = call "HEWH Find Header.vi"("Expression"=w152, "Header"=w120) -> ("Index"=w168:i32)  [unwired: 9 in]
      n46 = call "HEWH Find Header.vi"("Expression"=w151, "Header"=w120) -> ("Index"=w170:i32)  [unwired: 9 in]
      n47 = Search 1D Array(1D array=w120, element=w146) -> (index of element=w143:i32)  [unwired: 1 in]
      n48 = Search 1D Array(1D array=w120, element=w145) -> (index of element=w142:i32)  [unwired: 1 in]
      n49 = case shown="Default" w170 {
        selector: w170 -> [w189 _]
        tunnel: [w196 w199] -> w148
        tunnel: w144 -> [w195 w200]
        tunnel: w169 -> [w191 w198]
        tunnel: w168 -> [w190 w197]
        frame Default {
          n50 = Index Array(array=w195, index (col) #1=w191, index (col) #2=w190, index (col) #3=w189) -> (element #1=w194:dbl[], element #2=w193:dbl[], element #3=w192:dbl[])  [unwired: 3 in]
          n51 = Compound Arithmetic op=OR(w194, w193, w192) -> (w196:i32[])
        }
        frame -1 {
          n52 = Index Array(array=w200, index (col) #1=w198, index (col) #2=w197) -> (element #1=w202:dbl[], element #2=w201:dbl[])  [unwired: 2 in]
          n53 = Compound Arithmetic op=OR(w202, w201) -> (w199:i32[])
        }
      }
      n54 = Index Array(array=w144, index (col) #1=w176, index (col) #2=w177, index (col) #3=w178, index (col) #4=w179, index (col) #5=w180, index (col) #6=w181, index (col) #7=w166, index (col) #8=w165, index (col) #9=w164, index (col) #10=w171) -> (element #1=w187:dbl[], element #2=w182:dbl[], element #3=w183:dbl[], element #4=w184:dbl[], element #5=w185:dbl[], element #6=w186:dbl[], element #7=w175:dbl[], element #8=w174:dbl[], element #9=w173:dbl[], element #10=w172:dbl[])  [unwired: 10 in]
      n55 = Index Array(array=w144, index (col) #1=w143, index (col) #2=w142) -> (element #1=w141:dbl[], element #2=w140:dbl[])  [unwired: 2 in]
      n56 = Array Size(array=w148) -> (size(s)=w149:i32)
      n57 = Initialize Array(0.0, w149) -> (w147:dbl[])
      n58 = Build Array(w187, w182, w183, w184, w185, w186, w175, w174, w173, w172, w148, w147, w147, w147, w141, w140) -> (w188:dbl[][])
      n59 = Transpose 2D Array(2D array=w188) -> (transposed array=w167:dbl[][])
      n60 = Bundle By Name(cluster=w123, "Raw Data.Elapsed Time Index (DBL)"=0 ("Raw Data.Elapsed Time Index"), "Raw Data.Software Elapsed Time Index (DBL)"=1 ("Raw Data.Elapsed Time Index"), "Raw Data.TC Tree Avg Index (DBL)"=2 ("Raw Data.Elapsed Time Index"), "Raw Data.Watt Hours -Wh Index (DBL)"=3 ("Raw Data.Elapsed Time Index"), "Raw Data.Totalized Flow Index (DBL)"=4 ("Raw Data.Elapsed Time Index"), "Raw Data.Flow Rate Index (DBL)"=5 ("Raw Data.Elapsed Time Index"), "Raw Data.RTDin Index (DBL)"=6 ("Raw Data.Elapsed Time Index"), "Raw Data.RTDout Index (DBL)"=7 ("Raw Data.Elapsed Time Index"), "Raw Data.RTDamb Index (DBL)"=8 ("Raw Data.Elapsed Time Index"), "Raw Data.Energy BTU Index (DBL)"=9 ("Raw Data.Elapsed Time Index"), "Raw Data.Heat Source Index (DBL)"=10 ("Raw Data.Elapsed Time Index"), "Raw Data.Hot Water Rate GPM (DBL)"=11 ("Raw Data.Elapsed Time Index"), "Raw Data.Hot Water Total - GAL (DBL)"=12 ("Raw Data.Elapsed Time Index"), "Raw Data.Humidity -% RH (DBL)"=13 ("Raw Data.Elapsed Time Index"), "Raw Data.Voltage - V (DBL)"=14 ("Raw Data.Elapsed Time Index"), "Raw Data.Draw Count (DBL)"=15 ("Raw Data.Elapsed Time Index")) -> (w122:T1)
    }
    frame "CSA Inlet Side Meter" {
      # "Header"
      # "Consolidate heat source status. This \nallows for other labs to run through this\ncalculation (CSA)."
      n61 = Index Array(array=w204, index (row)=0) -> (element=w203:string[])  [unwired: 1 in]
      n62 = Search 1D Array(1D array=w203, element="Elapsed Time" ("regular expression")) -> (index of element=w224:i32)  [unwired: 1 in]
      n63 = Search 1D Array(1D array=w203, element="Mean Tank Temp" ("regular expression")) -> (index of element=w235:i32)  [unwired: 1 in]
      n64 = Search 1D Array(1D array=w203, element="Watt-Hours" ("regular expression")) -> (index of element=w234:i32)  [unwired: 1 in]
      n65 = Search 1D Array(1D array=w203, element="Total Water Cons. @Inlet" ("regular expression")) -> (index of element=w233:i32)  [unwired: 1 in]
      n66 = Search 1D Array(1D array=w203, element="Water Flow Rate @Inlet" ("regular expression")) -> (index of element=w232:i32)  [unwired: 1 in]
      n67 = Search 1D Array(1D array=w203, element="Inlet Temp" ("regular expression")) -> (index of element=w231:i32)  [unwired: 1 in]
      n68 = Search 1D Array(1D array=w203, element="Outlet Temp" ("regular expression")) -> (index of element=w230:i32)  [unwired: 1 in]
      n69 = Search 1D Array(1D array=w203, element="Ambient Temp" ("regular expression")) -> (index of element=w229:i32)  [unwired: 1 in]
      n70 = Search 1D Array(1D array=w203, element="Q Total" ("regular expression")) -> (index of element=w228:i32)  [unwired: 1 in]
      n71 = Search 1D Array(1D array=w203, element="Upper Element" ("regular expression")) -> (index of element=w227:i32)  [unwired: 1 in]
      n72 = Search 1D Array(1D array=w203, element="Burner/Lower Element" ("regular expression")) -> (index of element=w226:i32)  [unwired: 1 in]
      n73 = Index Array(array=w261, index (col) #1=w224, index (col) #2=w224, index (col) #3=w235, index (col) #4=w234, index (col) #5=w233, index (col) #6=w232, index (col) #7=w231, index (col) #8=w230, index (col) #9=w229, index (col) #10=w228, index (col) #11=w227, index (col) #12=w226) -> (element #1=w258:dbl[], element #2=w253:dbl[], element #3=w254:dbl[], element #4=w255:dbl[], element #5=w256:dbl[], element #6=w257:dbl[], element #7=w252:dbl[], element #8=w251:dbl[], element #9=w250:dbl[], element #10=w249:dbl[], element #11=w248:dbl[], element #12=w247:dbl[])  [unwired: 12 in]
      n74 = Compound Arithmetic op=OR(w248, w247) -> (w246:i32[])
      n75 = Build Array(w258, w253, w254, w255, w256, w257, w252, w251, w250, w249, w246) -> (w259:dbl[][])
      n76 = Transpose 2D Array(2D array=w259) -> (transposed array=w260:dbl[][])
      n77 = Bundle By Name(cluster=w207, "Raw Data.Elapsed Time Index (DBL)"=0 ("Raw Data.Elapsed Time Index"), "Raw Data.Software Elapsed Time Index (DBL)"=1 ("Raw Data.Elapsed Time Index"), "Raw Data.TC Tree Avg Index (DBL)"=2 ("Raw Data.Elapsed Time Index"), "Raw Data.Watt Hours -Wh Index (DBL)"=3 ("Raw Data.Elapsed Time Index"), "Raw Data.Totalized Flow Index (DBL)"=4 ("Raw Data.Elapsed Time Index"), "Raw Data.Flow Rate Index (DBL)"=5 ("Raw Data.Elapsed Time Index"), "Raw Data.RTDin Index (DBL)"=6 ("Raw Data.Elapsed Time Index"), "Raw Data.RTDout Index (DBL)"=7 ("Raw Data.Elapsed Time Index"), "Raw Data.RTDamb Index (DBL)"=8 ("Raw Data.Elapsed Time Index"), "Raw Data.Energy BTU Index (DBL)"=9 ("Raw Data.Elapsed Time Index"), "Raw Data.Heat Source Index (DBL)"=10 ("Raw Data.Elapsed Time Index"), "Raw Data.Hot Water Rate GPM (DBL)"=11 ("Raw Data.Elapsed Time Index"), "Raw Data.Hot Water Total - GAL (DBL)"=12 ("Raw Data.Elapsed Time Index"), "Raw Data.Humidity -% RH (DBL)"=13 ("Raw Data.Elapsed Time Index"), "Raw Data.Voltage - V (DBL)"=14 ("Raw Data.Elapsed Time Index"), "Raw Data.Draw Count (DBL)"=15 ("Raw Data.Elapsed Time Index")) -> (w206:T1)
    }
  }
  "UEF Calculated Values Input out" <- w25
  "Full Data DBL Out" <- w24
  "error out" <- "error in (no error)"
